vi "Wait for Server.vi"(2 "error in":errorcluster, 3 "vi reference in":refnum<vi>) -> (0 "error out":errorcluster, 1 "vi reference out":refnum<vi>)   [LabVIEW 2010]
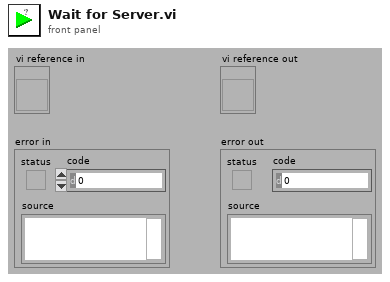
[diagram p1: front panel]
types:
  T1 = enum32{"Bad", "Idle", "Run top level", "Running"}
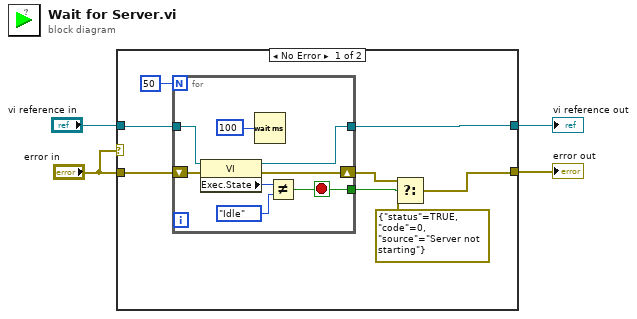
[diagram p0: block diagram]
diagram:
  n1 = case shown="No Error" "error in" {
    tunnel: "vi reference in" -> [w11 w22]
    tunnel: "error in" -> [w10 w21]
    tunnel: [w9 w22] -> w3
    tunnel: [w6 w21] -> w2
    frame No Error {
      n2 = for {
        N: 50 -> [_]
        tunnel: w11 -> [w20]
        shift-right: [w15] -> w7
        shift-left: w10 -> [w16]
        tunnel: [w14] -> w9
        tunnel: [w13] -> w8
        stop <- w13 stop-if-true
        n3 = property class="VI"(reference=w20, error in=w16) -> (reference out=w14:refnum<vi>, error out=w15:errorcluster, "Exec.State"=w19:T1)
        n4 = Wait (ms)(milliseconds to wait=u32 100) -> ()  [unwired: 1 out]
        n5 = Not Equal?(x=w19, y=T1."Idle") -> (x != y?=w13:bool)
      }
      n6 = Select(t=w7, s=w8, f=errorcluster {"status"=TRUE, "code"=0, "source"="Server not starting"}) -> (s? t:f=w6:errorcluster)
    }
    frame Error {
    }
  }
  "vi reference out" <- w3
  "error out" <- w2
